vi "SVD Factorization.vi"   [LabVIEW 2020, in "NI_AALPro.lvlib"]
doc: "Performs the singular value decomposition (SVD) of a given m-by-n matrix <B>A</B>. The dimentions of U, S, and V are m x min(m, n), min(m, n), and n x min(m, n), respectively."
uses:
  <vilib>/Analysis/NI_AALPro.lvlib
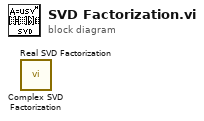
[diagram p0: block diagram]
diagram:
  n1 = call <vilib>:"Complex SVD Factorization.vi"() -> ()  [unwired: 1 in, 4 out]
  n2 = call <vilib>:"Real SVD Factorization.vi"() -> ()  [unwired: 1 in, 4 out]
